vi "tsdb_unload_lin_dbs.vi"(8 "error in (no error)":errorcluster caption="错误输入（无错误）", 11 "路径输入":path) -> (0 "error out":errorcluster caption="错误输出", 2 "function return":i32, 3 "路径输出":path)   [LabVIEW 2014]
doc: "Function Introduction :\nUninstall all loaded lin databases\nCall location :\ninput parameter :\nnothing\nReturn value :\n==0: Execution successful\nOther values: Query error code"
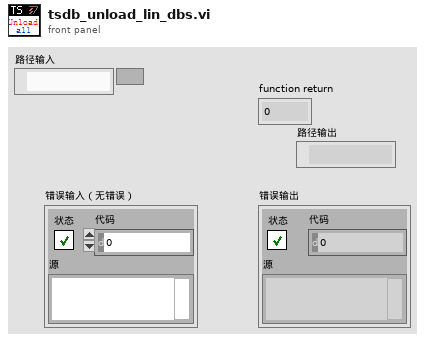
[diagram p1: front panel]
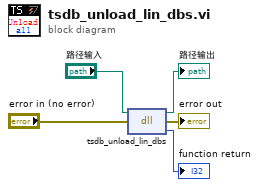
[diagram p0: block diagram]
diagram:
  n1 = dll-call lib="D:/Work/LabVIEW Code/TSMaster Labview SDK/LabVIEW/LabVIEW-TSMasterAPI_CLN/TSMasterAPI_LabVIEW-2024-08-27 16-32-25/Not_organized_vi/TSMaster.*" fn="tsdb_unload_lin_dbs"(path in="路径输入", error in="error in (no error)") -> (path out=→"路径输出":path, error out=→"error out":errorcluster, "返回类型"=→"function return":i32)  [unwired: 1 in]
